vi "Wiimote Parse Acceleration.vi"(8 "error in":errorcluster, 11 "pReportBuffer in":u8[](array[numeric]) format="%02x") -> (0 "error out":errorcluster, 3 "Wiimote Acceleration Raw out":T1)   [LabVIEW 2011, in "Wiimote.lvlib"]
uses:
  Wiimote Acceleration.ctl
  Wiimote.lvlib
panel:
  in  "Wiimote Acceleration in":T1
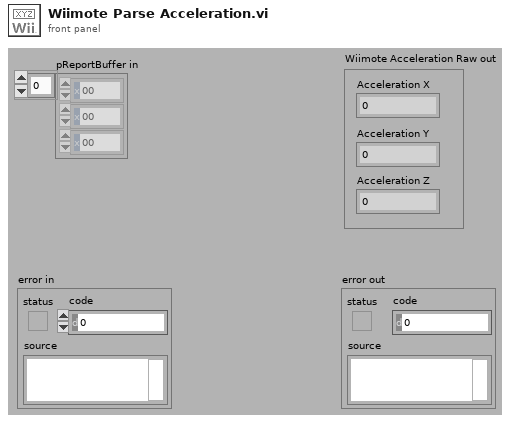
[diagram p1: front panel]
types:
  T1 = typedef "Wiimote.lvlib/Wiimote Acceleration.ctl" = cluster{"Acceleration X":dbl, "Acceleration Y":dbl, "Acceleration Z":dbl}
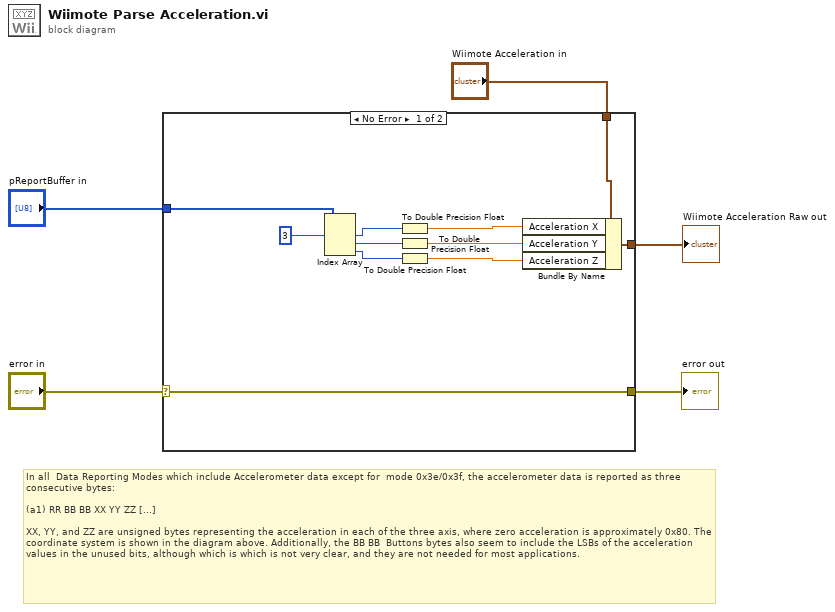
[diagram p0: block diagram]
diagram:
  # "In all  Data Reporting Modes which include Accelerometer data except for  mode 0x3e/0x3f, the accelerometer data is reported as three consecutive bytes:\n\n(a1) RR BB BB XX YY ZZ [...]\n\nXX, YY, and ZZ are unsigned bytes representing the acceleration in each of the three axis, where zero acceleration is approximately 0x80. The coordinate system is shown in the diagram above. Additionally, the BB BB  Buttons bytes also seem to include the LSBs of the acceleration values in the unused bits, although which is which is not very clear, and they are not needed for most applications."
  n1 = case shown="No Error" "error in" {
    selector: "error in" -> [w16 w17]
    tunnel: [w16 w17] -> w4
    tunnel: "pReportBuffer in" -> [w11 _]
    tunnel: "Wiimote Acceleration in" -> [w10 _]
    tunnel: [w9 _] -> w1
    frame No Error {
      n2 = Index Array(array=w11, index #1=3 ("index")) -> (element #1=w13:u8, element #2=w14:u8, element #3=w15:u8)  [unwired: 2 in]
      n3 = To Double Precision Float(number=w13) -> (double precision float=w8:dbl)
      n4 = To Double Precision Float(number=w14) -> (double precision float=w7:dbl)
      n5 = To Double Precision Float(number=w15) -> (double precision float=w6:dbl)
      n6 = Bundle By Name(cluster=w10, "Acceleration X"=w8, "Acceleration Y"=w7, "Acceleration Z"=w6) -> (w9:T1)
    }
    frame Error {
    }
  }
  "error out" <- w4
  "Wiimote Acceleration Raw out" <- w1
